vi "Energia Create Build Cpp Command.vi"(10 "input filename":path, 11 "Arduino IDE installation directory":path) -> (3 "String":string)   [LabVIEW 2014]
uses:
  <vilib>/regexp/Match Regular Expression.xnode
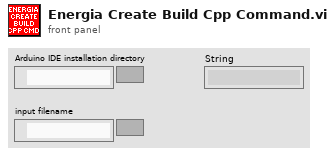
[diagram p1: front panel]
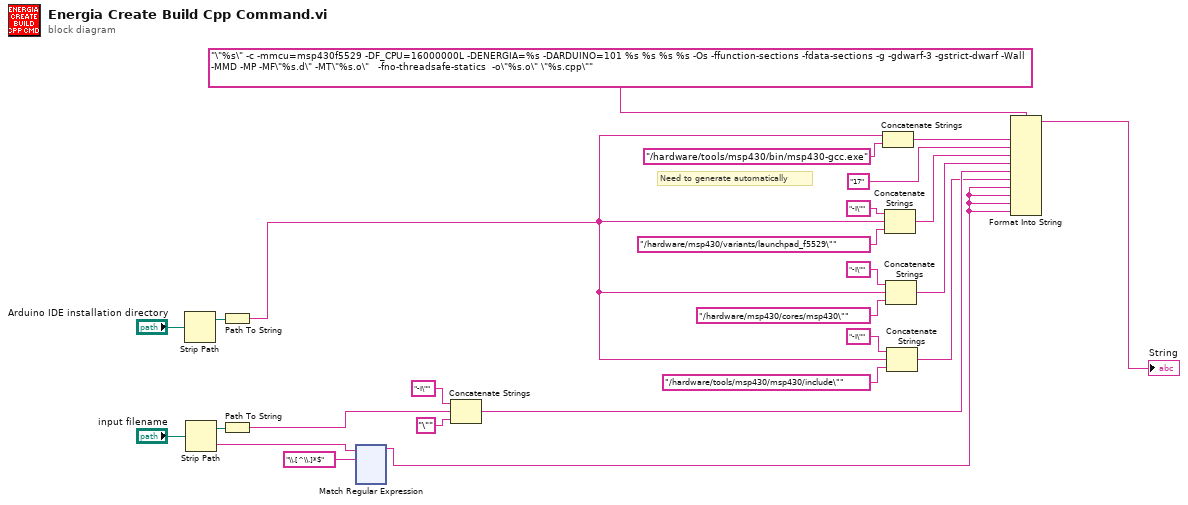
[diagram p0: block diagram]
diagram:
  # "Need to generate automatically"
  n1 = Strip Path(path="Arduino IDE installation directory") -> (stripped path=w3:path)  [unwired: 1 out]
  n2 = Strip Path(path="input filename") -> (stripped path=w11:path, name=w25:string)
  n3 = Path To String(path=w3) -> (string=w15:string)
  n4 = Path To String(path=w11) -> (string=w23:string)
  n5 = xnode "Match Regular Expression"("input string"=w25, "regular expression"="\\.[^\\.]*$" ("input string")) -> ("before match"=w26:string)  [unwired: 4 in, 4 out]
  n6 = Concatenate Strings("-I\"" ("format string"), w23, "\"" ("format string")) -> (w21:string)
  n7 = Concatenate Strings(w15, "/hardware/tools/msp430/bin/msp430-gcc.exe" ("format string")) -> (w16:string)
  n8 = Concatenate Strings("-I\"" ("format string"), w15, "/hardware/msp430/variants/launchpad_f5529\"" ("format string")) -> (w18:string)
  n9 = Concatenate Strings("-I\"" ("format string"), w15, "/hardware/msp430/cores/msp430\"" ("format string")) -> (w19:string)
  n10 = Concatenate Strings("-I\"" ("format string"), w15, "/hardware/tools/msp430/msp430/include\"" ("format string")) -> (w20:string)
  n11 = Format Into String(format string="\"%s\" -c -mmcu=msp430f5529 -DF_CPU=16000000L -DENERGIA=%s -DARDUINO=101 %s %s %s %s -Os -ffunction-sections -fdata-sections -g -gdwarf-3 -gstrict-dwarf -Wall -MMD -MP -MF\"%s.d\" -MT\"%s.o\"   -fno-threadsafe-statics  -o\"%s.o\" \"%s.cpp\"", w16, "17" ("format string"), w18, w19, w21, w20, w26, w26, w26, w26) -> (resulting string=→"String":string)  [unwired: 2 in, 1 out]
